vi "Refresh Rooms Status.vi"(0 "Rooms Manager Model in":refnum<class "Rooms Manager Model.lvclass">, 5 "Rooms List":T2[](array[typedef]), 7 "Room Size Details":T1[](array[typedef]), 11 "error in (no error)":errorcluster) -> (4 "Rooms Manager Model out":refnum<class "Rooms Manager Model.lvclass">, 15 "error out":errorcluster)   [LabVIEW 2023, in "Rooms Manager Model.lvlib" / "Rooms Manager Model.lvclass"]
uses:
  Rooms Manager Model.lvclass
  Central Data Manager/Central Data Manager/Room Details.ctl
  Central Data Manager/Central Data Manager/Room Occupancy Status.ctl
  Central Data Manager/Central Data Manager/Guest Details.ctl
  Central Data Manager/Central Data Manager/Room Size Details.ctl
  Rooms Manager UI/Rooms Manager UI/Room Details.ctl
  Rooms Manager Model.lvclass/Rooms Manager Model.ctl
  Rooms Manager UI/Rooms Manager UI Messages/Refresh Rooms Status Msg/Refresh Rooms Status Msg.lvclass/Refresh Rooms Status Msg.ctl
  <vilib>/ActorFramework/Message Enqueuer/Message Enqueuer.lvclass/Message Enqueuer.ctl
  <vilib>/ActorFramework/Message Enqueuer/Enqueue.vi
  Rooms Manager UI/Rooms Manager UI Messages/Refresh Rooms Status Msg/Refresh Rooms Status Msg.lvclass
  C:/Program Files/National Instruments/LabVIEW 2023/vi.lib/ActorFramework/Message/Message.lvclass
  <vilib>/ActorFramework/Message Priority Queue/Priority Enqueue.vi
  Rooms Manager UI/Rooms Manager UI/Rooms Manager UI.lvclass
  Central Data Manager/Central Data Manager/Central Data Manager.lvclass
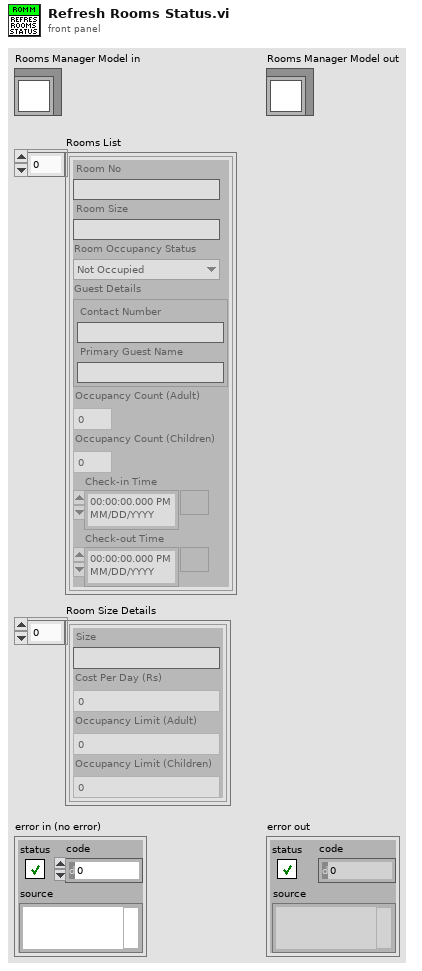
[diagram p1: front panel]
types:
  T1 = typedef "Central Data Manager.lvlib/Central Data Manager.lvclass/Room Size Details.ctl" = cluster{"Size":string, "Cost Per Day (Rs)":u32, "Occupancy Limit (Adult)":u32, "Occupancy Limit (Children)":u32}
  T2 = typedef "Central Data Manager.lvlib/Central Data Manager.lvclass/Room Details.ctl" = cluster{"Room No":string, "Room Size":string, "Room Occupancy Status":T3, "Guest Details":T4, "Occupancy Count (Adult)":u32, "Occupancy Count (Children)":u32, "Check-in Time":timestamp, "Check-out Time":timestamp}
  T3 = typedef "Central Data Manager.lvlib/Central Data Manager.lvclass/Room Occupancy Status.ctl" = enum16{"Not Occupied", "Occupied", "Under Maintainance", "Not Servicable"}
  T4 = typedef "Central Data Manager.lvlib/Central Data Manager.lvclass/Guest Details.ctl" = cluster{"Contact Number":string, "Primary Guest Name":string}
  T5 = typedef "Rooms Manager UI.lvlib/Rooms Manager UI.lvclass/Room Details.ctl" = cluster{"Room No":string, "Occupied":bool, "Alert":bool, "Maintainance":bool}
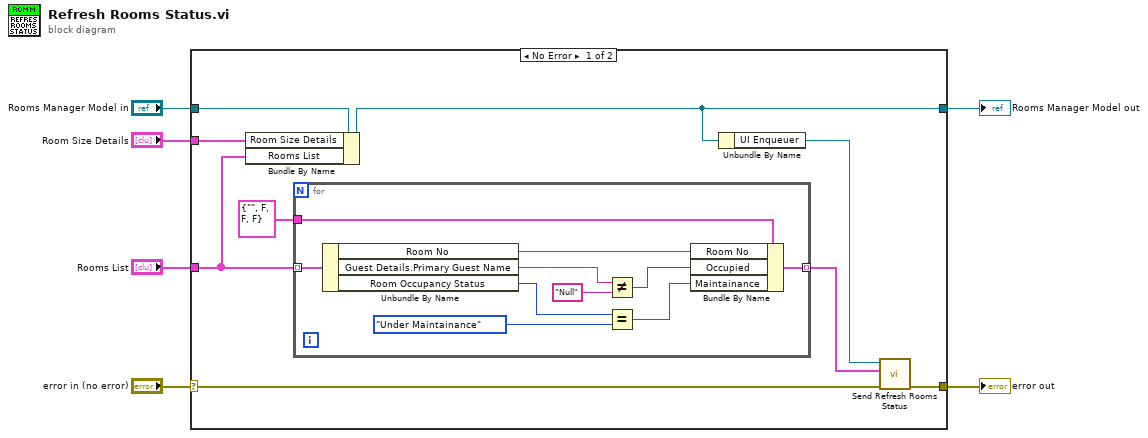
[diagram p0: block diagram]
diagram:
  n1 = case shown="No Error" "error in (no error)" {
    selector: "error in (no error)" -> [w15 w27]
    tunnel: [w14 w27] -> w5
    tunnel: [w9 w26] -> w3
    tunnel: "Rooms Manager Model in" -> [w13 w26]
    tunnel: "Rooms List" -> [w8 _]
    tunnel: "Room Size Details" -> [w7 _]
    frame No Error {
      n2 = Bundle By Name(cluster=w13, "Room Size Details"=w7, "Rooms List"=w8) -> (w9:refnum<class "Rooms Manager Model.lvclass">)
      n3 = for {
        tunnel: w8 -> [w25] mode=indexing
        tunnel: T5 {"Room No"="", "Occupied"=FALSE, "Alert"=FALSE, "Maintainance"=FALSE} ("Room Details") -> [w24]
        tunnel: [w16] -> w10 mode=indexing
        n4 = Unbundle By Name(w25) -> ("Room No"=w23:string, "Guest Details.Primary Guest Name"=w22:string, "Room Occupancy Status"=w20:T3)
        n5 = Not Equal?(x=w22, y="Null") -> (x != y?=w18:bool)
        n6 = Equal?(x=w20, y=Room_Occupancy_Status."Under Maintainance") -> (x = y?=w17:bool)
        n7 = Bundle By Name(cluster=w24, "Room No"=w23, "Occupied"=w18, "Maintainance"=w17) -> (w16:T5)
      }
      n8 = Unbundle By Name(w9) -> ("UI Enqueuer"=w12:refnum<class "Message Enqueuer.lvclass">)
      n9 = call "Send Refresh Rooms Status.vi"("error in (no error)"=w15, "Room Details"=w10, "Message Enqueuer"=w12) -> ("error out"=w14:errorcluster)  [unwired: 7 in, 1 out]
    }
    frame Error {
    }
  }
  "error out" <- w5
  "Rooms Manager Model out" <- w3
